vi "target-detection.vi"() -> ()   [LabVIEW 2013]
uses:
  <vilib>/Rock Robotics/WPI/Camera/WPI_CameraSettings Read MJPG.ctl
  <vilib>/Rock Robotics/WPI/Camera/WPI_CameraImageSize.ctl
  <vilib>/vision/NI_Vision_Development_Module.lvlib
panel:
  out "Thresholded":T1(plugin-control)
  out "Camera Raw":T1(plugin-control)
  in  "Aspect Ratio Upper Bound":dbl format="%#_13g"
  in  "Rectangularity Cutoff":dbl format="%#_13g"
  in  "Aspect Ratio Lower Bound":dbl format="%#_13g"
  in  "Area Cutoff":dbl format="%#_13g"
  in  "Blue Range":cluster{"Lower value":i32, "Upper value":i32}={"Lower value"=0, "Upper value"=255}
  in  "Green Range":cluster{"Lower value":i32, "Upper value":i32}={"Lower value"=70, "Upper value"=255}
  in  "Red Range":cluster{"Lower value":i32, "Upper value":i32}={"Lower value"=0, "Upper value"=255}
  out "Target Detected":bool
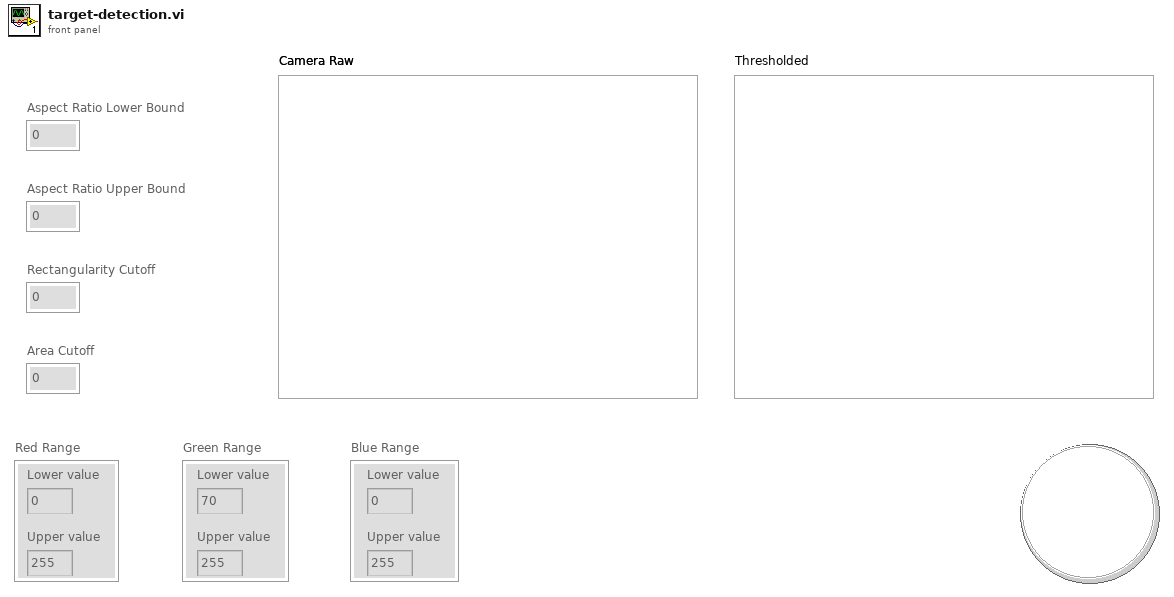
[diagram p1: front panel]
types:
  T1 = typedef "IMAQ Image.ctl" = refnum<image>
  T2 = typedef "Image Type" = u32
  T3 = typedef "WPI_CameraSettings Read MJPG.ctl" = cluster{"fps":i32, "compression":i32, "Image Size":T4}
  T4 = typedef "WPI_CameraImageSize.ctl" = enum16{"640x480", "320x240", "160x120"}
  T5 = typedef "Particle Parameters" = i32
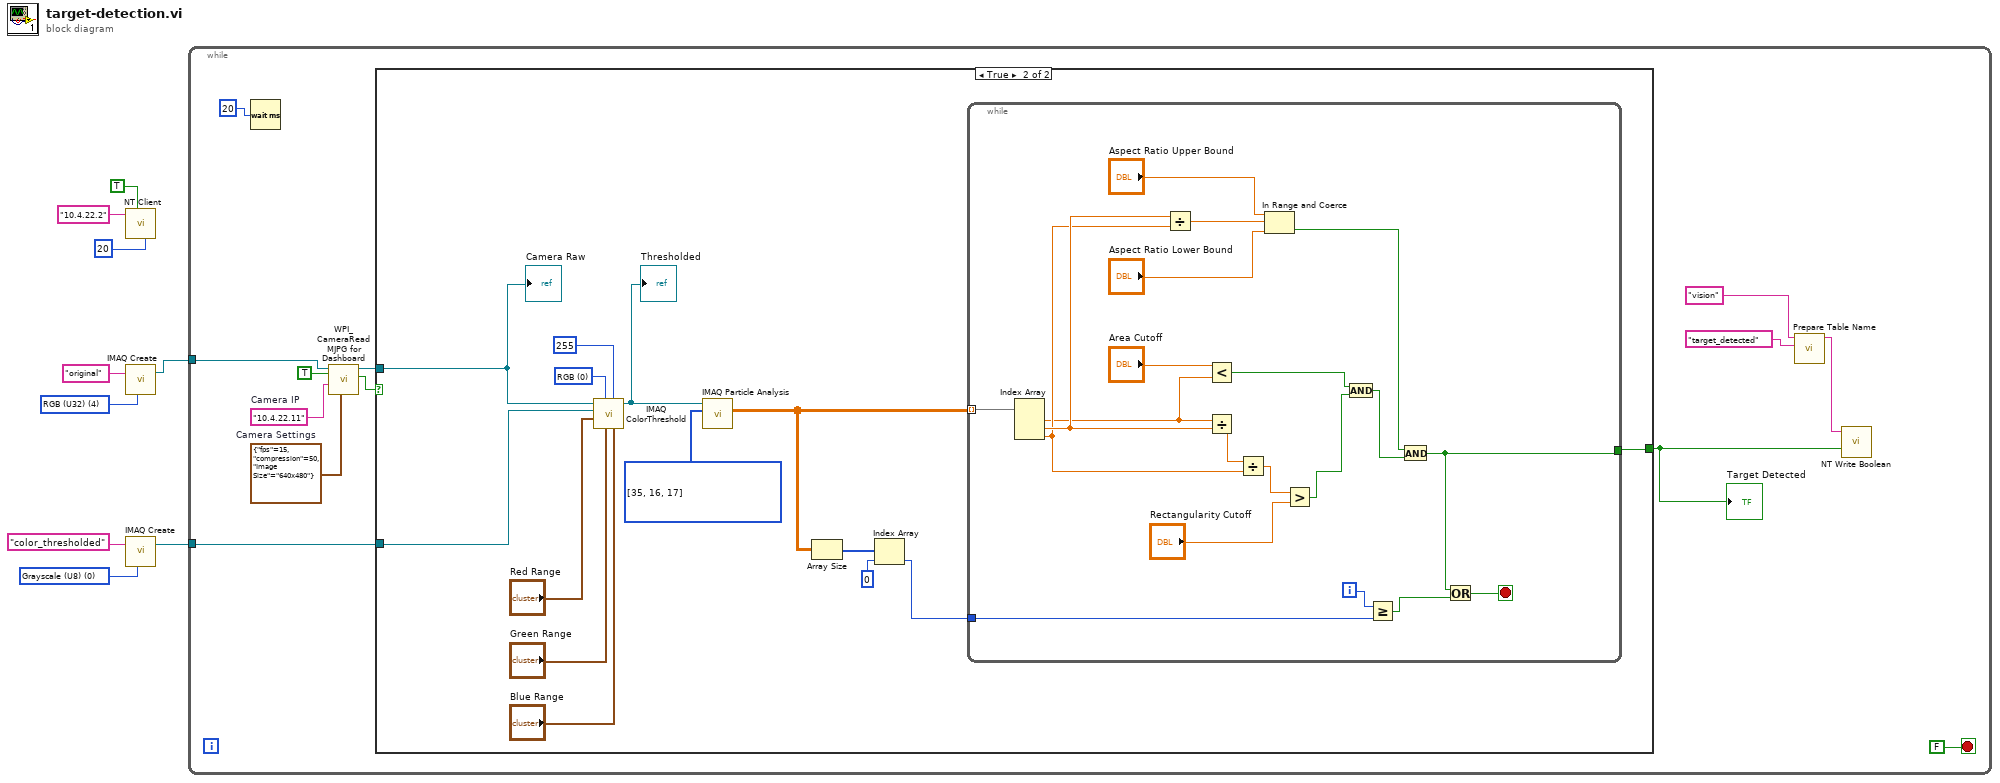
[diagram p0: block diagram]
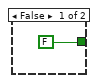
[diagram p2: hidden frame]
diagram:
  w5 = T2 0 items=["Grayscale (U8)", "Grayscale (I16)", "Grayscale (SGL)", "Complex (CSG)", "RGB (U32)", "HSL (U32)", "RGB (U64)", "Grayscale (U16)"] ("Image Type")
  w8 = T2 4 items=["Grayscale (U8)", "Grayscale (I16)", "Grayscale (SGL)", "Complex (CSG)", "RGB (U32)", "HSL (U32)", "RGB (U64)", "Grayscale (U16)"] ("Image Type")
  n1 = call <vilib>:"NT Client.vi"("Update Time"=20, "Automatic restart"=TRUE, "Server IP Address"="10.4.22.2") -> ()  [unwired: 9 in]
  n2 = call "IMAQ Create"("Image Name"="original", "Image Type"=w8) -> ("New Image"=w7:T1)  [unwired: 3 in, 1 out]
  n3 = call "IMAQ Create"("Image Name"="color_thresholded", "Image Type"=w5) -> ("New Image"=w4:T1)  [unwired: 3 in, 1 out]
  n4 = while {
    tunnel: w7 -> [w20]
    tunnel: w4 -> [w19]
    stop <- FALSE stop-if-true
    w17 = T3 {"fps"=15, "compression"=50, "Image Size"=enum."640x480"}  # Camera Settings
    w22 = "10.4.22.11"  # Camera IP
    n5 = Wait (ms)(milliseconds to wait=u32 20) -> ()  [unwired: 1 out]
    n6 = call <vilib>:"WPI_CameraRead MJPG for Dashboard.vi"("Camera Settings"=w17, "Camera IP"=w22, "Enable"=TRUE, "Refnum in"=w20) -> ("Active"=w10:bool, "Refnum out"=w15:T1)  [unwired: 4 in, 2 out]
    n7 = case shown="True" w10 {
      tunnel: w19 -> [_ w37]
      tunnel: [FALSE w36] -> w18
      tunnel: w15 -> [_ w35]
      frame False {
      }
      frame True {
        w30 = T5[] [35, 16, 17] items=["Center of Mass X", "Center of Mass Y", "First Pixel X", "First Pixel Y", "Bounding Rect Left", "Bounding Rect Top", "Bounding Rect Right", "Bounding Rect Bottom", "Max Feret Diameter Start X", "Max Feret Diameter Start Y", "Max Feret Diameter End X", "Max Feret Diameter End Y", "Max Horiz. Segment Length Left", "Max Horiz. Segment Length Right", "Max Horiz. Segment Length Row", "-", "Bounding Rect Width", "Bounding Rect Height", "Bounding Rect Diagonal", "Perimeter", "Convex Hull Perimeter", "Holes' Perimeter", "Max Feret Diameter", "Equivalent Ellipse Major Axis", "Equivalent Ellipse Minor Axis", "Equivalent Ellipse Minor Axis (Feret)", "Equivalent Rect Long Side", "Equivalent Rect Short Side", "Equivalent Rect Diagonal", "Equivalent Rect Short Side (Feret)", "Average Horiz. Segment Length", "Average Vert. Segment Length", "Hydraulic Radius", "Waddel Disk Diameter", "-", "Area", "Holes' Area", "Particle & Holes' Area", "Convex Hull Area", "Image Area", "-", "Number of Holes", "Number of Horiz. Segments", "Number of Vert. Segments", "-", "Orientation", "Max Feret Diameter Orientation", "-", "% Area/Image Area", "% Area/(Particle & Holes' Area)", "Ratio of Equivalent Ellipse Axes", "Ratio of Equivalent Rect Sides", "-", "Elongation Factor", "Compactness Factor", "Heywood Circularity Factor", "Type Factor", "-", "Sum X", "Sum Y", "Sum XX", "Sum XY", "Sum YY", "Sum XXX", "Sum XXY", "Sum XYY", "Sum YYY", "-", "Moment of Inertia XX", "Moment of Inertia XY", "Moment of Inertia YY", "Moment of Inertia XXX", "Moment of Inertia XXY", "Moment of Inertia XYY", "Moment of Inertia YYY", "Norm. Moment of Inertia XX", "Norm. Moment of Inertia XY", "Norm. Moment of Inertia YY", "Norm. Moment of Inertia XXX", "Norm. Moment of Inertia XXY", "Norm. Moment of Inertia XYY", "Norm. Moment of Inertia YYY", "Hu Moment 1", "Hu Moment 2", "Hu Moment 3", "Hu Moment 4", "Hu Moment 5", "Hu Moment 6", "Hu Moment 7"] ("Pixel Measurements")
        w34 = u16 0 items=["RGB", "HSL", "HSV", "HSI"] ("Color Mode")
        n8 = call "IMAQ ColorThreshold"("Blue or Luma or Val or Inten Range"="Blue Range", "Replace Value"=255, "Green or Sat Range"="Green Range", "Color Mode"=w34, "Red or Hue Range"="Red Range", "Image Dst"=w37, "Image Src"=w35) -> ("Image Dst Out"=w25:T1)  [unwired: 3 in, 1 out]
        "Thresholded" <- w25
        n9 = call "IMAQ Particle Analysis"("Pixel Measurements"=w30, "Image"=w25) -> ("Particle Measurements (Pixels)"=w29:dbl[][])  [unwired: 4 in, 5 out]
        n10 = Array Size(array=w29) -> (size(s)=w28:i32[])
        n11 = Index Array(array=w28, index=0) -> (element=w26:i32)
        n12 = while {
          tunnel: w29 -> [w54] mode=indexing
          tunnel: w26 -> [w47]
          tunnel: [w44] -> w36
          i -> [w48]
          stop <- w45 stop-if-true
          n13 = Index Array(array=w54) -> (element #1=w40:dbl, element #2=w53:dbl, element #3=w52:dbl)  [unwired: 3 in]
          n14 = Divide(x=w53, y=w52) -> (x/y=w51:dbl)
          n15 = Less?(x="Area Cutoff", y=w40) -> (x < y?=w39:bool)
          n16 = Divide(x=w40, y=w53) -> (x/y=w57:dbl)
          n17 = Divide(x=w57, y=w52) -> (x/y=w56:dbl)
          n18 = In Range and Coerce(upper limit="Aspect Ratio Upper Bound", x=w51, lower limit="Aspect Ratio Lower Bound") -> (In Range?=w50:bool)  [unwired: 1 out]
          n19 = Greater?(x=w56, y="Rectangularity Cutoff") -> (0:w55:bool)
          n20 = And(x=w39, y=w55) -> (x .and. y?=w49:bool)
          n21 = Greater Or Equal?(x=w48, y=w47) -> (x >= y?=w46:bool)
          n22 = And(x=w50, y=w49) -> (x .and. y?=w44:bool)
          n23 = Or(x=w44, y=w46) -> (x .or. y?=w45:bool)
        }
        "Camera Raw" <- w35
      }
    }
    "Target Detected" <- w18
    n24 = call <vilib>:"Prepare Table Name.vi"("Name"="target_detected", "Table Prefix"="vision") -> ("Prefixed Name"=w14:string)  [unwired: 9 in]
    n25 = call <vilib>:"NT Write Boolean.vi"("Boolean"=w18, "Name"=w14) -> ()  [unwired: 9 in, 1 out]
  }
